vi "SendMessageCluster.vi"(6 "timeout in ms (-1)":i32=-1, 7 "priority (-1, highest)":i32=-1, 8 "error in":errorcluster, 10 "message":T1, 11 "queues in":refnum<class "CLM_PriorityLocalMessage.lvclass">) -> (0 "error out":errorcluster, 1 "priority used":i32, 3 "queues out":refnum<class "CLM_PriorityLocalMessage.lvclass">, 4 "timed out?":bool)   [LabVIEW 2013, in "CLM_PriorityLocalMessage.lvclass"]
uses:
  CLM_PriorityLocalMessage.lvclass
  LocalMessage/Message.ctl
  CLM_PriorityLocalMessage.lvclass/CLM_PriorityLocalMessage.ctl
  LocalMessage_Queue/CLM_LocalMessage_Queue.lvclass/CLM_LocalMessage_Queue.ctl
  LocalMessage_Queue/CLM_LocalMessage_Queue.lvclass
  LocalMessage/CLM_LocalMessage.lvclass
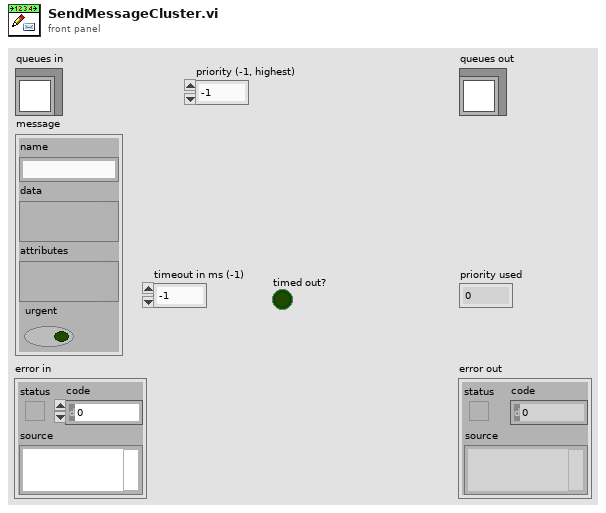
[diagram p1: front panel]
types:
  T1 = typedef "CLM_LocalMessage.lvclass/Message.ctl" = cluster{"name":string, "data":variant, "attributes":variant, "urgent":bool}
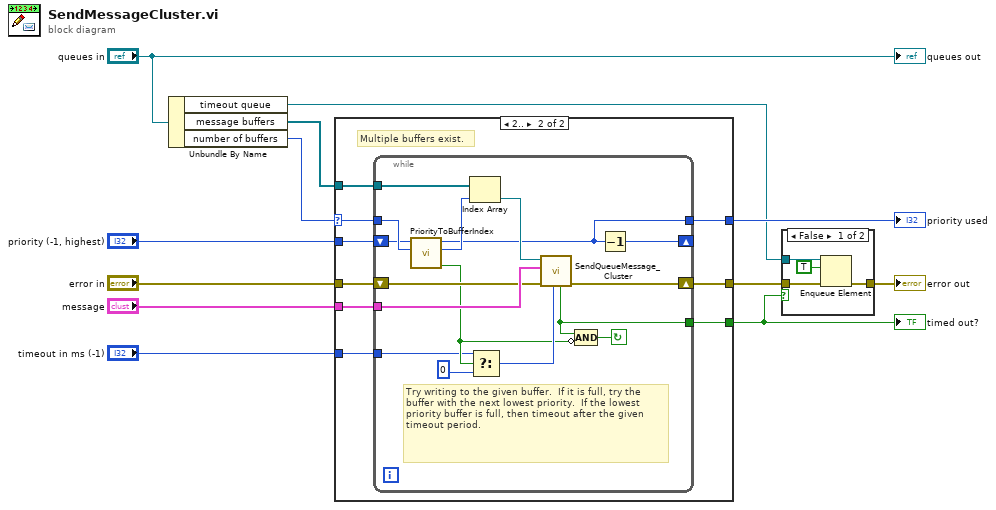
[diagram p0: block diagram]
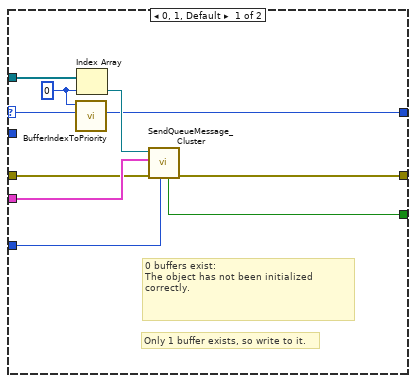
[diagram p2: hidden frame]
diagram:
  n1 = Unbundle By Name("queues in") -> ("timeout queue"=w2:refnum<queue>, "message buffers"=w7:refnum<class "CLM_LocalMessage_Queue.lvclass">[], "number of buffers"=w1:i32)
  n2 = case shown="2.." w1 {
    selector: w1 -> [w14 w23]
    tunnel: "priority (-1, highest)" -> [_ w24]
    tunnel: "message" -> [w20 w31]
    tunnel: "timeout in ms (-1)" -> [w18 w30]
    tunnel: "error in" -> [w19 w29]
    tunnel: w7 -> [w22 w28]
    tunnel: [w16 w27] -> w6
    tunnel: [w17 w26] -> w4
    tunnel: [w13 w25] -> w3
    frame 0, 1, Default {
      w15 = 0
      # "0 buffers exist:\nThe object has not been initialized correctly."
      # "Only 1 buffer exists, so write to it."
      n3 = call "BufferIndexToPriority.vi"("number of buffers"=w14, "buffer index"=w15) -> ("priority"=w13:i32)  [unwired: 6 in, 3 out]
      n4 = Index Array(array=w22, index=w15) -> (element=w21:refnum<class "CLM_LocalMessage_Queue.lvclass">)
      n5 = call "SendQueueMessage_Cluster.vi"("timeout in ms (-1)"=w18, "error in"=w19, "message"=w20, "message ref in"=w21) -> ("error out"=w16:errorcluster, "timed out?"=w17:bool)  [unwired: 5 in, 1 out]
    }
    frame 2.. {
      # "Multiple buffers exist."
      n6 = while {
        tunnel: w31 -> [w47]
        tunnel: w30 -> [w33]
        tunnel: [w41] -> w26
        tunnel: w28 -> [w44]
        shift-right: [w38] -> _
        shift-left: w24 -> [w37]
        shift-right: [w45] -> w27
        shift-left: w29 -> [w46]
        tunnel: [w34] -> w25
        tunnel: w23 -> [w39]
        stop <- w40 continue-if-true
        # "Try writing to the given buffer.  If it is full, try the buffer with the next lowest priority.  If the lowest priority buffer is full, then timeout after the given timeout period."
        n7 = call "PriorityToBufferIndex.vi"("number of buffers"=w39, "priority"=w37) -> ("lowest priority?"=w36:bool, "buffer index"=w35:i32, "priority out"=w34:i32)  [unwired: 6 in, 1 out]
        n8 = Index Array(array=w44, index=w35) -> (element=w43:refnum<class "CLM_LocalMessage_Queue.lvclass">)
        n9 = Select(t=w33, s=w36, f=0 ("timeout in ms (-1)")) -> (s? t:f=w42:i32)
        n10 = call "SendQueueMessage_Cluster.vi"("timeout in ms (-1)"=w42, "error in"=w46, "message"=w47, "message ref in"=w43) -> ("error out"=w45:errorcluster, "timed out?"=w41:bool)  [unwired: 5 in, 1 out]
        n11 = Compound Arithmetic op=AND(w41, invert w36) -> (w40:bool)
        n12 = Decrement(x=w34) -> (x-1=w38:i32)
      }
    }
  }
  "timed out?" <- w4
  "priority used" <- w3
  n13 = case shown="False" w4 {
    tunnel: w6 -> [w51 w52]
    tunnel: [w50 w52] -> w5
    tunnel: w2 -> [w49 _]
    frame False {
      n14 = Enqueue Element(queue=w49, element=TRUE, error in (no error)=w51) -> (error out=w50:errorcluster)  [unwired: 1 in, 2 out]
    }
    frame True {
    }
  }
  "error out" <- w5
  "queues out" <- "queues in"
